vi "MeasurementType.Edit.vi"(7 "Max Shots":T1(ring)=enum."1", 8 "error in (no error)":errorcluster, 9 "Stages":string[](array[string])=["Boost", "Battery", "Off"], 11 "Item Ref in":T2 format="%.0x") -> (0 "error out":errorcluster)   [LabVIEW 2019, in "Fuel Injector Analysis Addon System Explorer.lvlib"]
uses:
  Fuel Injector Analysis Addon System Explorer.lvlib
  <vilib>/NI VeriStand/Custom Device API/Custom Device Item Ref.ctl
  Addon Shared/SubVIs/Constants.vi
  <vilib>/NI VeriStand/Custom Device API/Get Item Property (Path).vi
  Addon Shared/Fuel Injector Analysis Addon Shared.lvlib
  <vilib>/NI VeriStand/Custom Device API/Custom Device API.lvlib
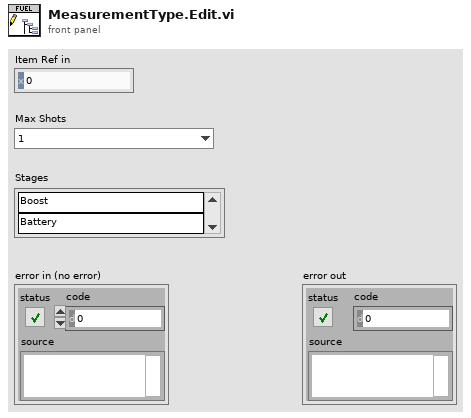
[diagram p1: front panel]
types:
  T1 = enum16{"0", "1", "2", "3", "4", "5", "6", "7", "8"}
  T2 = typedef "Custom Device API.lvlib/Custom Device Item Ref.ctl" = u64
  T3 = typedef "Custom Device API.lvlib/Custom Device Item Info.ctl" = cluster{"Name":string, "Is Channel":bool, "GUID":string, "Is Waveform":bool}
  T4 = typedef "Fifo_DMA_Config.ctl" = cluster{"Name":string, "Depth":u32, "Write? (Deprecated:Use Implementation)":bool, "Physical Channel":u32, "Base Address":u32, "Data Width":u32, "Data Type":T5, "FXP Properties":variant, "Write Window Address":u32, "Implementation":T6, "Control Set":u32}
  T5 = typedef "niFpgaDataTypeControl.ctl" = enum32{"Boolean", "I8", "I16", "I32", "I64", "U8", "U16", "U32", "U64", "FXP", "CustomControl", "SGL"}
  T6 = typedef "niFpgaDmaChannelImplementation.ctl" = enum16{"niFpgaTargetToHost", "niFpgaHostToTarget", "niFpgaPeerToPeerWriter", "niFpgaPeerToPeerReader", "niCoreTargetToHost", "niCoreHostToTarget"}
  T7 = typedef "niFpgaBitfileStructure_VI.ctl" = cluster{"Name":string, "RegisterMap":T8[], "Icon":T13}
  T8 = typedef "nirviControlStructure.ctl" = cluster{"Name":string, "Hidden":bool, "Indicator":bool, "Flattened Type":string, "Grouping":cluster{"Grouped":bool, "Member Names":string[], "Member IDs":u32[]}, "Address":u32, "Size":u32, "Class":u32, "Internal":bool, "Typedef":T9, "ID":u32, "Bidirectional":bool, "Synchronous":bool, "Mechanical Action":T10, "Sub Controls":T11[], "Access May Timeout":bool, "Register Node":bool}
  T9 = typedef "nirviTypdefDescription.ctl" = cluster{"Typedef":bool, "Path":path}
  T10 = typedef "nirviMechanicalAction.ctl" = enum8{"Switch When Pressed", "Switch When Released", "Switch Until Released", "Latch When Pressed", "Latch When Released", "Latch Until Released"}
  T11 = typedef "nirviSubControlStructure.ctl" = cluster{"Name":string, "flattened Type":string, "Cluster Information":T12, "Typedef":T9}
  T12 = typedef "nirviClusterElementControl.ctl" = cluster{"Name Hierarchy":string[], "Item Order":u32[]}
  T13 = typedef "imagedata.ctl" = cluster{"image type":i32, "image depth":i32, "image":u8[], "mask":u8[], "colors":u32[], "Rectangle":cluster{"left":i16, "top":i16, "right":i16, "bottom":i16}}
  T14 = typedef "Fuel Injector Analysis Addon Shared.lvlib/Register.Info.ctl" = cluster{"Name":string, "Data Type":T15, "Default Value":variant}
  T15 = typedef "Fuel Injector Analysis Addon Shared.lvlib/FPGA Data Types.ctl" = enum8{"<Null>", "Injector.Core.Setting", "Injector.Global.Setting", "Injector.Mux.Setting", "Injector.Timing"}
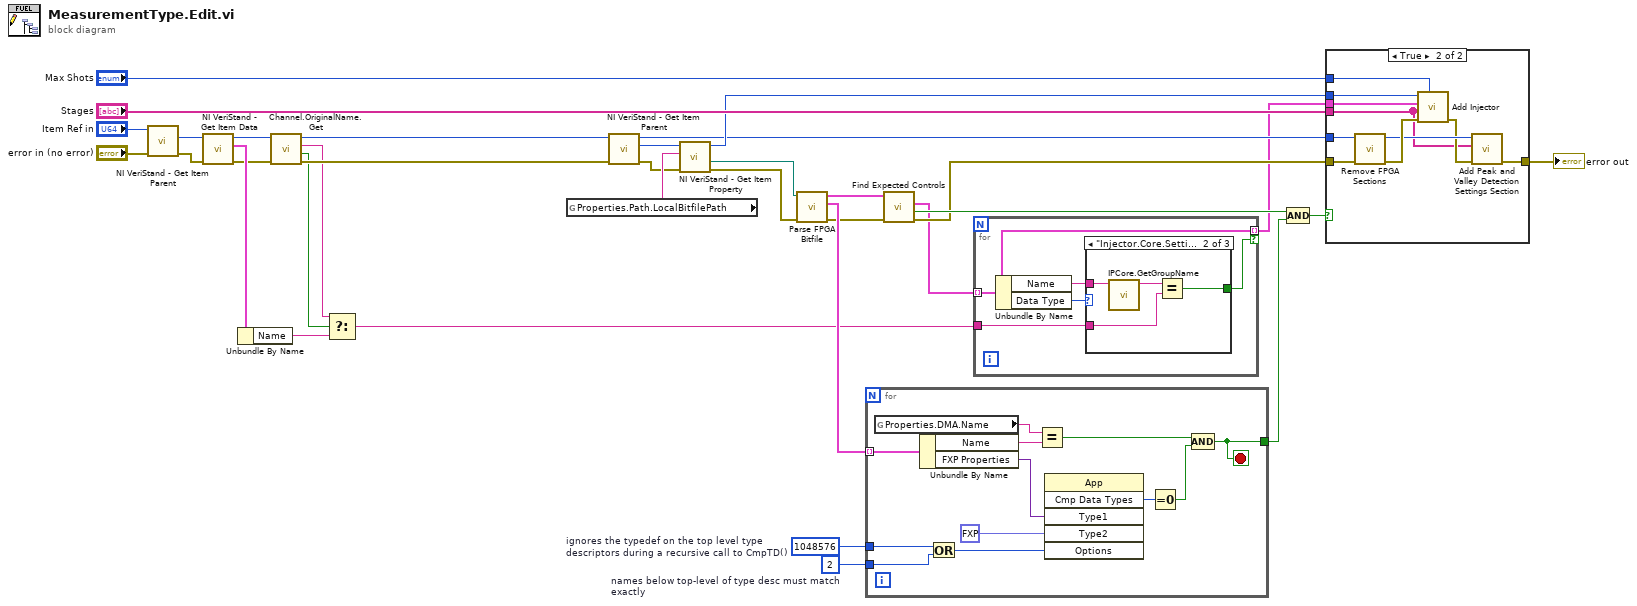
[diagram p0: block diagram]
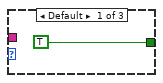
[diagram p2: hidden frame]
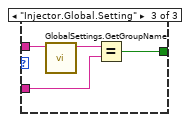
[diagram p3: hidden frame]
diagram:
  w30 = 2  # names below top-level of type desc must match exactly
  w31 = 1048576  # ignores the typedef on the top level type descriptors during a recursive call to CmpTD()
  n1 = call <vilib>:"NI VeriStand - Get Item Parent.vi"("error in (no error)"="error in (no error)", "Item Ref in"="Item Ref in") -> ("error out"=w11:errorcluster, "Parent Ref"=w19:T2)  [unwired: 6 in, 2 out]
  n2 = call <vilib>:"NI VeriStand - Get Item Data.vi"("error in (no error)"=w11, "Item Ref in"=w19) -> ("error out"=w8:errorcluster, "Item Info"=w12:T3, "Item Ref out"=w6:T2)  [unwired: 6 in, 1 out]
  n3 = Unbundle By Name(w12) -> ("Name"=w2:string)
  n4 = call "Channel.OriginalName.Get.vi"("error in (no error)"=w8, "Ref in"=w6) -> ("error out"=w7:errorcluster, "Found?"=w4:bool, "Value"=w3:string, "Ref out"=w5:T2)  [unwired: 6 in]
  n5 = Select(t=w3, s=w4, f=w2) -> (s? t:f=w1:string)
  n6 = global read "Constants.vi" "Properties.Path.LocalBitfilePath"() -> (w20:string)
  n7 = call <vilib>:"NI VeriStand - Get Item Parent.vi"("error in (no error)"=w7, "Item Ref in"=w5) -> ("error out"=w17:errorcluster, "Parent Ref"=w18:T2, "Item Ref out"=w13:T2)  [unwired: 6 in, 1 out]
  n8 = call-poly <vilib>:"NI VeriStand - Get Item Property.vi"("error in (no error)"=w17, "Property Name"=w20, "Item Ref in"=w18) -> ("error out"=w15:errorcluster, "Value"=w14:path, "Item Ref out"=w16:T2)  [unwired: 5 in, 1 out]
  n9 = call "Parse FPGA Bitfile.vi"("error in (no error)"=w15, "Path"=w14) -> ("error out"=w23:errorcluster, "DMA configuration array"=w25:T4[], "vi info"=w24:T7)  [unwired: 7 in]
  n10 = for {
    tunnel: w25 -> [w46] mode=indexing
    tunnel: [w42] -> w27
    tunnel: w31 -> [w37]
    tunnel: w30 -> [w36]
    stop <- w42 stop-if-true
    n11 = global read "Constants.vi" "Properties.DMA.Name"() -> (w44:string)
    n12 = Unbundle By Name(w46) -> ("Name"=w45:string, "FXP Properties"=w35:variant)
    n13 = Or(x=w37, y=w36) -> (x .or. y?=w41:i32)
    n14 = Equal?(x=w44, y=w45) -> (x = y?=w43:bool)
    n15 = invoke class="App" method="Cmp Data Types"("Type1"=w35, "Type2"=fxp<+/-,32,8> 0.0, "Options"=w41) -> ("Compare Data Types"=w39:i32)  [unwired: 3 in, 5 out]
    n16 = Equal To 0?(x=w39) -> (x = 0?=w38:bool)
    n17 = Compound Arithmetic op=AND(w43, w38) -> (w42:bool)
  }
  n18 = call "Find Expected Controls.vi"("error in"=w23, "vi info"=w24) -> ("error out"=w22:errorcluster, "Use?"=w26:bool, "Controls"=w10:T14[])  [unwired: 5 in, 2 out]
  n19 = for {
    tunnel: w10 -> [w49] mode=indexing
    tunnel: [w49] -> w9 mode=indexing if=w47
    tunnel: w1 -> [w48]
    n20 = Unbundle By Name(w49) -> ("Name"=w50:string, "Data Type"=w51:T15)
    n21 = case shown="\"Injector.Core.Setting\"" w51 {
      tunnel: w50 -> [_ w56 w60]
      tunnel: [TRUE w53 w57] -> w47
      tunnel: w48 -> [_ w55 w59]
      frame Default {
      }
      frame "Injector.Core.Setting" {
        n22 = call "IPCore.GetGroupName.vi"("Name"=w56) -> ("Group"=w54:string)  [unwired: 10 in]
        n23 = Equal?(x=w54, y=w55) -> (x = y?=w53:bool)
      }
      frame "Injector.Global.Setting" {
        n24 = call "GlobalSettings.GetGroupName.vi"("Name"=w60) -> ("Group"=w58:string)  [unwired: 10 in]
        n25 = Equal?(x=w58, y=w59) -> (x = y?=w57:bool)
      }
    }
  }
  n26 = Compound Arithmetic op=AND(w26, w27) -> (w21:bool)
  n27 = case shown="True" w21 {
    tunnel: w13 -> [_ w67]
    tunnel: w22 -> [w61 w68]
    tunnel: [w61 w63] -> w34
    tunnel: w9 -> [_ w70]
    tunnel: "Stages" -> [_ w62]
    tunnel: "Max Shots" -> [_ w69]
    tunnel: w16 -> [_ w66]
    frame False {
    }
    frame True {
      n28 = call "Remove FPGA Sections.vi"("error in (no error)"=w68, "Item Ref in"=w67) -> ("error out"=w71:errorcluster, "Item Ref out"=w65:T2)  [unwired: 8 in]
      n29 = call "Add Injector.vi"("Max Shots"=w69, "error in (no error)"=w71, "Stages"=w62, "Controls"=w70, "Item Ref"=w66) -> ("error out"=w64:errorcluster)  [unwired: 5 in, 1 out]
      n30 = call "Add Peak and Valley Detection Settings Section.vi"("error in (no error)"=w64, "Stages"=w62, "Global Settings Item Ref in"=w65) -> ("error out"=w63:errorcluster)  [unwired: 7 in, 1 out]
    }
  }
  "error out" <- w34
